vi "TransmintFrame.vi"(7 "Hex and Dec":bool, 8 "error in (no error)":errorcluster, 10 "data":T1[](array[typedef]) {"event ID" format="%x"; "payload" format="%x"; "timestamp" format="%<%.7X\n%x>T"; "type" items=["LIN Data"=64, "LIN Bus Error"=65, "LIN No Response"=66, "Delay"=224, "Log Trigger"=225, "Start Trigger"=226]; "identifier" format="%x"}) -> (0 "error out":errorcluster, 1 "DataByte":string[](array[string]), 2 "Output Array":string[][](array[string]))   [LabVIEW 2018]
uses:
  <vilib>/xnet/xnet.llb/XNET Frame LIN.ctl
  <vilib>/xnet/xnet.llb/XNET Frame Type LIN.ctl
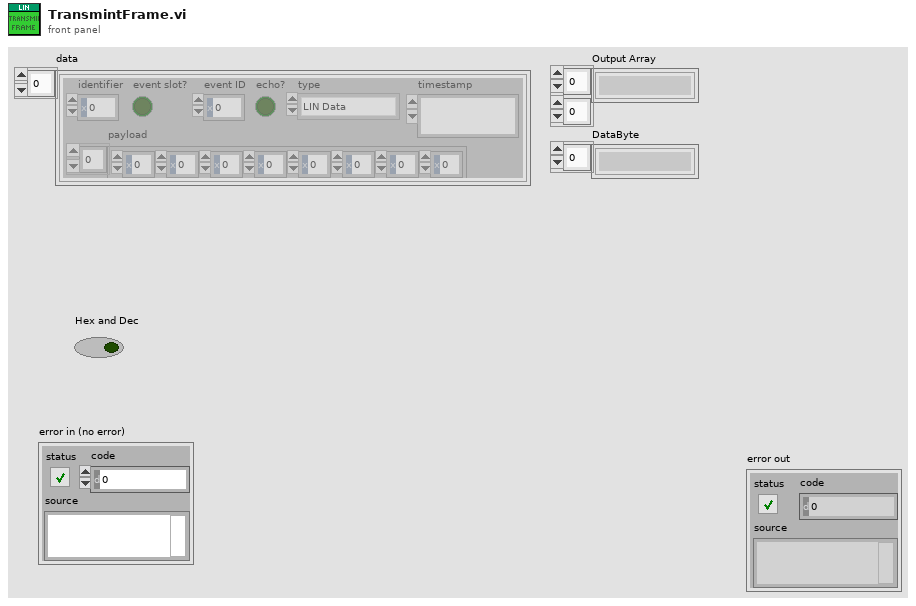
[diagram p1: front panel]
types:
  T1 = typedef "XNET Frame LIN.ctl" = cluster{"timestamp":timestamp, "payload":u8[], "identifier":u32, "type":T2, "event ID":u8, "event slot?":bool, "echo?":bool}
  T2 = typedef "XNET Frame Type LIN.ctl" = u8
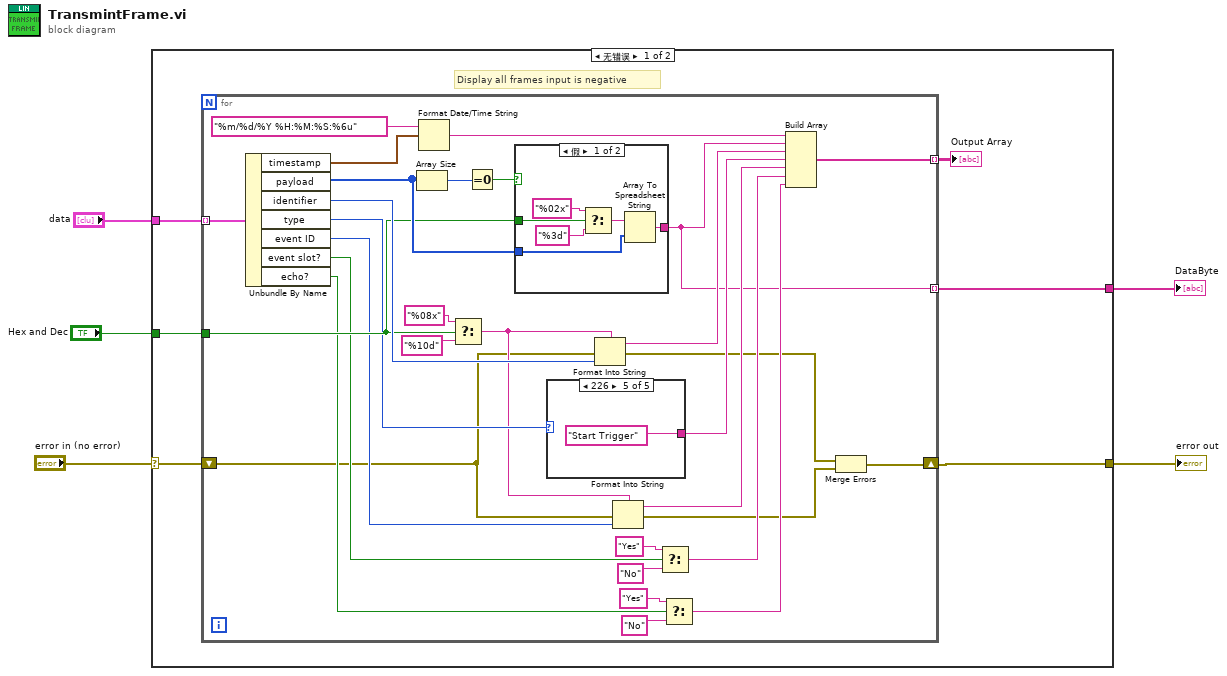
[diagram p0: block diagram]
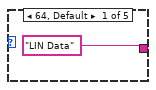
[diagram p2: hidden frame]
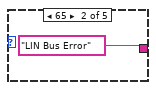
[diagram p3: hidden frame]
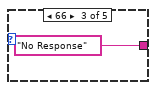
[diagram p4: hidden frame]
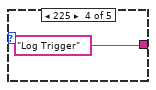
[diagram p5: hidden frame]
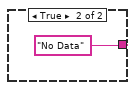
[diagram p6: hidden frame]
diagram:
  n1 = case shown="无错误" "error in (no error)" {
    selector: "error in (no error)" -> [w7 w55]
    tunnel: "data" -> [w11 _]
    tunnel: "Hex and Dec" -> [w10 _]
    tunnel: [w8 _] -> w2
    tunnel: [w6 w55] -> w1
    frame No Error {
      # "Display all frames input is negative"
      n2 = for {
        tunnel: w11 -> [w42] mode=indexing
        tunnel: w10 -> [w35]
        tunnel: [w17] -> w9 mode=indexing
        tunnel: [w16] -> w8 mode=indexing
        shift-right: [w12] -> w6
        shift-left: w7 -> [w15]
        n3 = Unbundle By Name(w42) -> ("timestamp"=w41:timestamp, "payload"=w37:u8[], "identifier"=w36:u32, "type"=w30:T2, "event ID"=w27:u8, "event slot?"=w23:bool, "echo?"=w20:bool)
        n4 = Array Size(array=w37) -> (size(s)=w39:i32)
        n5 = Format Date/Time String(time format string (%c)="%m/%d/%Y %H:%M:%S:%6u", seconds (now)=w41) -> (date/time string=w32:string)  [unwired: 1 in]
        n6 = Select(t="%08x", s=w35, f="%10d") -> (s? t:f=w28:string)
        n7 = Equal To 0?(x=w39) -> (x = 0?=w38:bool)
        n8 = case shown="假" w38 {
          tunnel: w35 -> [w53 _]
          tunnel: w37 -> [w49 _]
          tunnel: [w48 "No Data"] -> w16
          frame False {
            n9 = Select(t="%02x", s=w53, f="%3d") -> (s? t:f=w50:string)
            n10 = Array To Spreadsheet String(array=w49, 3:w50) -> (spreadsheet string=w48:string)  [unwired: 1 in]
          }
          frame True {
          }
        }
        n11 = case shown="226" w30 {
          tunnel: ["LIN Data" "LIN Bus Error" "No Response" "Log Trigger" "Start Trigger"] -> w29
          frame 64, Default {
          }
          frame 65 {
          }
          frame 66 {
          }
          frame 225 {
          }
          frame 226 {
          }
        }
        n12 = Format Into String(format string=w28, error in=w15, w36) -> (resulting string=w31:string, error out=w14:errorcluster)  [unwired: 1 in]
        n13 = Format Into String(format string=w28, error in=w15, w27) -> (resulting string=w26:string, error out=w13:errorcluster)  [unwired: 1 in]
        n14 = Select(t="Yes", s=w23, f="No") -> (s? t:f=w19:string)
        n15 = Select(t="Yes", s=w20, f="No") -> (s? t:f=w18:string)
        n16 = Build Array(w32, w16, w31, w29, w26, w19, w18) -> (w17:string[])
        n17 = Merge Errors(w14, w13) -> (w12:errorcluster)
      }
      "Output Array" <- w9
    }
    frame Error {
    }
  }
  "error out" <- w1
  "DataByte" <- w2
